vi "Can软件版本号.vi"() -> (3 "软件版本号":string)   [LabVIEW 2020]
uses:
  Global_Variable/Global.vi
  Libraries/ZLG_CAN/ZLG_CAN.lvlib
  Libraries/S7/S7.lvlib
panel:
  in  "波特率":u32(ring)=11 items=["5Kbps", "10Kbps", "20Kbps", "40Kbps", "50Kbps", "80Kbps", "100Kbps", "125Kbps", "200Kbps", "250Kbps", "400Kbps", "500Kbps", "666Kbps", "800Kbps", "1000Kbps"]
  in  "索引":u32(ring) items=["0", "1", "2", "3", "4", "5", "6", "7", "8"]
  in  "设备类型":u32(ring)=27 items=["PCI5121"=1, "PCI9810"=2, "USBCAN1"=3, "USBCAN2"=4, "PCI9820"=5, "PCI5110"=7, "PC104CAN"=11, "CANETUDP"=12, "PCI9840B"=14, "PC104C2"=15, "PCI9820I"=16, "CANETTCP"=17, "PCIE9221"=24, "PCI5010U"=19, "USBCAN_E_U"=20, "USBCAN_2E_U"=21, "PCI5020U"=22, "PCIE9120I"=27, "PCIE9110I"=28, "PCIE9140I"=29]
  in  "CAN 通道":u32(ring) items=["0", "1"]
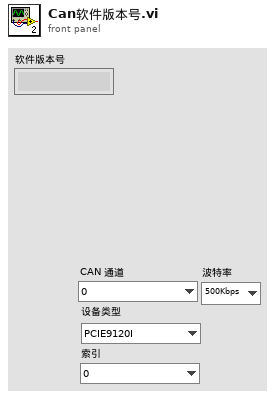
[diagram p1: front panel]
types:
  T1 = typedef "ZLG_CAN.lvlib/CAN_Frame.ctl" = cluster{"[0]":u8, "[1]":u8, "[2]":u8, "[3]":u8, "[4]":u8, "[5]":u8, "[6]":u8, "[7]":u8}
  T2 = typedef "ZLG_CAN.lvlib/Sent_Recive (Reply Payload)--cluster.ctl" = cluster{"Receive":T3[], "Sent_Recive_error":errorcluster}
  T3 = typedef "ZLG_CAN.lvlib/CAN_OBJ_R.ctl" = cluster{"ID":u32, "TimeStamp":u32, "TimeFlag":u8, "SendType":u8, "RemoteFlag":u8, "ExternFlag":u8, "DataLen":u8, "数值":u8, "数值":u8, "数值":u8, "数值":u8, "数值":u8, "数值":u8, "数值":u8, "数值":u8, "数值":u8, "数值":u8, "数值":u8}
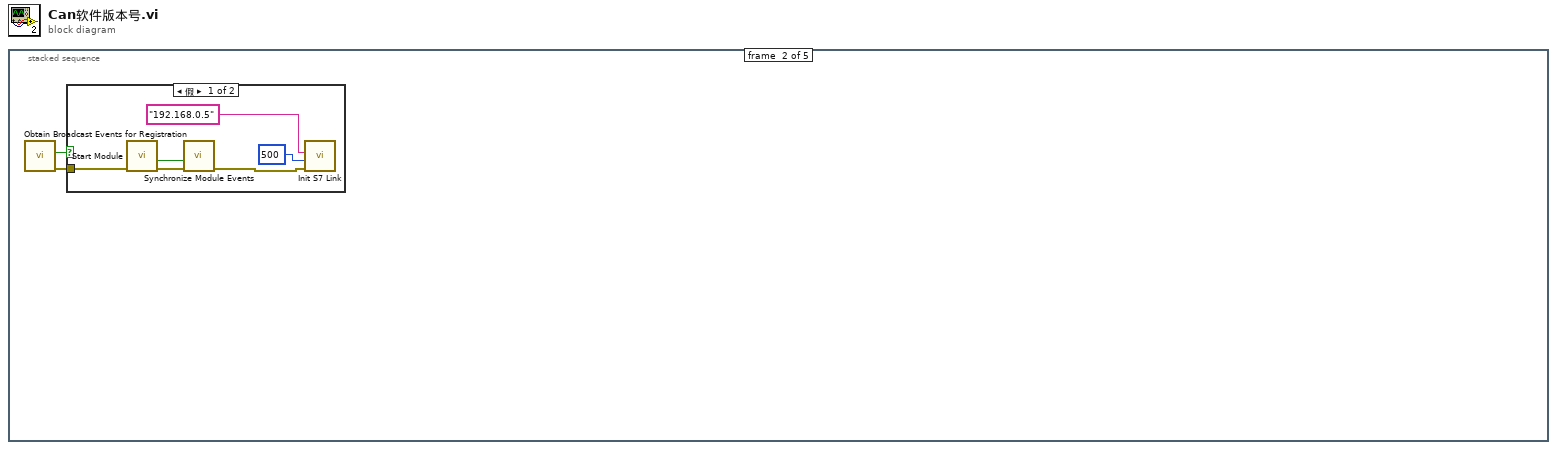
[diagram p0: block diagram]
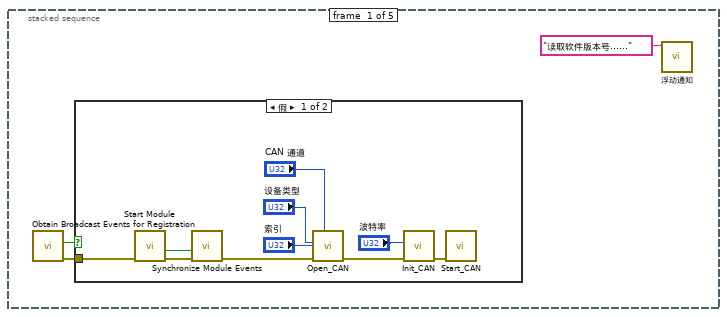
[diagram p2: hidden frame]
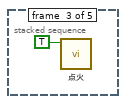
[diagram p5: hidden frame]
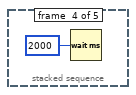
[diagram p6: hidden frame]
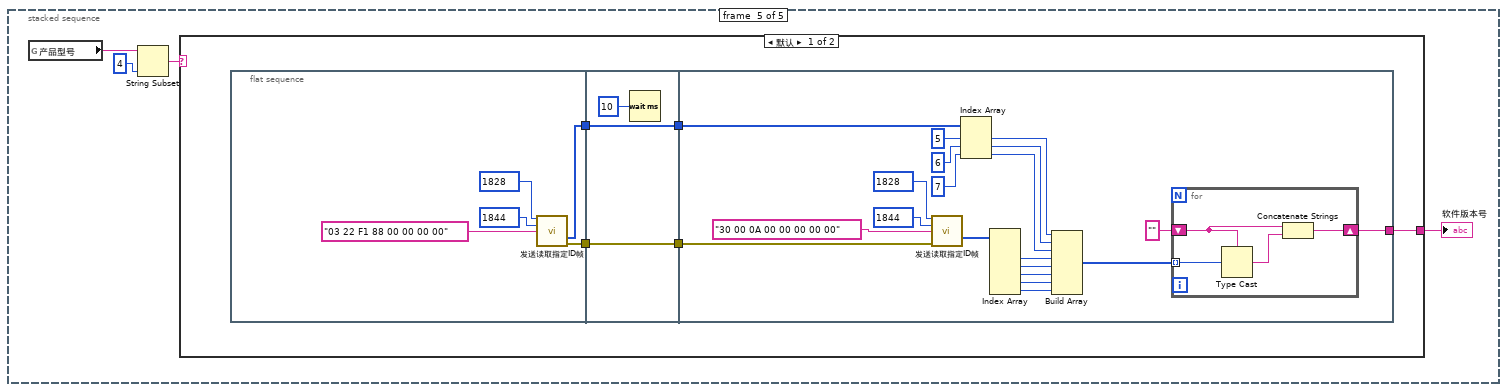
[diagram p7: hidden frame]
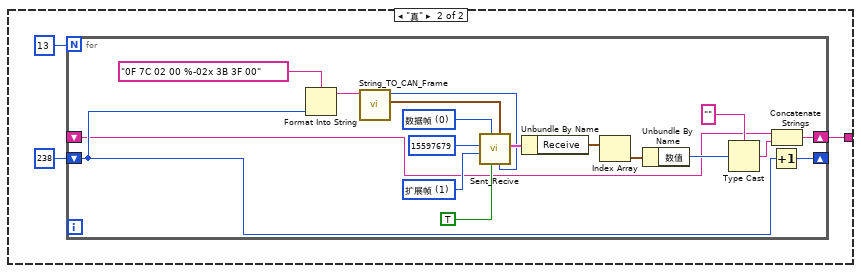
[diagram p8: hidden frame]
diagram:
  n1 = stacked-sequence {
    frame #0 {
      n2 = call "Obtain Broadcast Events for Registration.vi"() -> ("error out"=w2:errorcluster, "Already running?"=w3:bool)  [unwired: 9 in, 1 out]
      n3 = case shown="假" w3 {
        tunnel: w2 -> [w8 _]
        frame False {
          n4 = call "Start Module.vi"("error in (no error)"=w8) -> ("error out"=w9:errorcluster, "Wait for Event Sync?"=w10:bool)  [unwired: 7 in, 2 out]
          n5 = call "Synchronize Module Events.vi"("error in (no error)"=w9, "Wait for Event Sync?"=w10) -> ("error out"=w11:errorcluster)  [unwired: 9 in]
          n6 = call "Open_CAN.vi"("CAN 通道"="CAN 通道", "error in (no error)"=w11, "索引"="索引", "设备类型"="设备类型") -> ("error out"=w12:errorcluster)  [unwired: 7 in]
          n7 = call "Init_CAN.vi"("error in (no error)"=w12, "波特率"="波特率") -> ("error out"=w13:errorcluster)  [unwired: 9 in]
          n8 = call "Start_CAN.vi"("error in (no error)"=w13) -> ()  [unwired: 8 in, 3 out]
        }
        frame True {
        }
      }
      n9 = call "浮动通知.vi"("通知内容"="读取软件版本号……") -> ()  [unwired: 11 in]
    }
    frame #1 {
      n10 = call "Obtain Broadcast Events for Registration.vi"() -> ("error out"=w14:errorcluster, "Already running?"=w15:bool)  [unwired: 9 in, 1 out]
      n11 = case shown="假" w15 {
        tunnel: w14 -> [w16 _]
        frame False {
          n12 = call "Start Module.vi"("error in (no error)"=w16) -> ("error out"=w20:errorcluster, "Wait for Event Sync?"=w19:bool)  [unwired: 7 in, 2 out]
          n13 = call "Synchronize Module Events.vi"("error in (no error)"=w20, "Wait for Event Sync?"=w19) -> ("error out"=w21:errorcluster)  [unwired: 9 in]
          n14 = call "Init S7 Link.vi"("error in (no error)"=w21, "超时"=500, "IP"="192.168.0.5") -> ()  [unwired: 8 in, 1 out]
        }
        frame True {
        }
      }
    }
    frame #2 {
      n15 = call "点火.vi"("点火"=TRUE) -> ()  [unwired: 10 in, 1 out]
    }
    frame #3 {
      n16 = Wait (ms)(milliseconds to wait=u32 2000 ("等待时间（毫秒）")) -> ()  [unwired: 1 out]
    }
    frame #4 {
      n17 = global read "Global.vi" "产品型号"() -> (w26:string)
      n18 = String Subset(string=w26, length (rest)=4 ("长度（剩余）")) -> (substring=w24:string)  [unwired: 1 in]
      n19 = case shown="默认" w24 {
        tunnel: [w28 w65] -> w27
        frame Default {
          n20 = flat-sequence {
            tunnel: [w37] -> w32
            tunnel: [w33] -> w31
            tunnel: w32 -> [w40]
            tunnel: w31 -> [w39]
            tunnel: [w40] -> w30
            tunnel: [w39] -> w29
            tunnel: w30 -> [w45]
            tunnel: w29 -> [w46]
            tunnel: [w41] -> w28
            frame #0 {
              n21 = call "发送读取指定ID帧.vi"("T_ID"=u32 1828, "R_ID"=u32 1844 ("T_ID"), "CAN_Frame"="03 22 F1 88 00 00 00 00") -> ("Recive"=w37:u8[], "error out"=w33:errorcluster)  [unwired: 8 in, 3 out]
            }
            frame #1 {
              n22 = Wait (ms)(milliseconds to wait=u32 10 ("等待时间（毫秒）")) -> ()  [unwired: 1 out]
            }
            frame #2 {
              n23 = call "发送读取指定ID帧.vi"("T_ID"=u32 1828, "R_ID"=u32 1844 ("T_ID"), "CAN_Frame"="30 00 0A 00 00 00 00 00", "error in (no error)"=w46) -> ("Recive"=w60:u8[])  [unwired: 7 in, 4 out]
              n24 = Index Array(array=w45, index #1=5 ("索引"), index #2=6 ("索引"), index #3=7 ("索引")) -> (element #1=w59:u8, element #2=w58:u8, element #3=w57:u8)
              n25 = Index Array(array=w60) -> (element #2=w56:u8, element #3=w55:u8, element #4=w54:u8, element #5=w53:u8, element #6=w52:u8)  [unwired: 6 in, 1 out]
              n26 = Build Array(w59, w58, w57, w56, w55, w54, w53, w52) -> (w51:u8[])
              n27 = for {
                tunnel: w51 -> [w64] mode=indexing
                shift-right: [w61] -> w41
                shift-left: "" -> [w63]
                n28 = Type Cast(type=w63, x=w64) -> (*(type *) &x=w62:string)
                n29 = Concatenate Strings(w63, w62) -> (w61:string)
              }
            }
          }
        }
        frame "真" {
          n30 = for {
            N: 13 -> [_]
            shift-right: [w78] -> _
            shift-left: u8 238 -> [w79]
            shift-right: [w69] -> w65
            shift-left: _ -> [w68]
            w84 = u8 1 items=["标准帧", "扩展帧"] ("帧类型")
            w85 = u8 0 items=["数据帧", "远程帧"] ("帧格式")
            n31 = Format Into String(format string="0F 7C 02 00 %-02x 3B 3F 00" ("格式字符串"), w79) -> (resulting string=w81:string)  [unwired: 2 in, 1 out]
            n32 = call "String_TO_CAN_Frame.vi"("CAN_Frame"=w81) -> ("CAN_FRAME"=w77:T1, "DATA_LEN"=w76:i32)  [unwired: 9 in]
            n33 = call "Sent_Recive.vi"("帧长度"=w76, "CAN_FRAME"=w77, "wait for reply (T)"=TRUE, "帧格式"=w85, "帧类型"=w84, "ID"=u32 15597679) -> ("Reply Payload"=w82:T2)  [unwired: 3 in, 2 out]
            n34 = Unbundle By Name(w82) -> ("Receive"=w75:T3[])
            n35 = Index Array(array=w75) -> (element=w74:T3)  [unwired: 1 in]
            n36 = Unbundle By Name(w74) -> ("数值"=w72:u8)
            n37 = Type Cast(type="", x=w72) -> (*(type *) &x=w71:string)
            n38 = Increment(x=w79) -> (x+1=w78:u8)
            n39 = Concatenate Strings(w68, w71) -> (w69:string)
          }
        }
      }
      "软件版本号" <- w27
    }
  }
